vi "Find PS3 Controller.vi"(8 "error in (no error)":errorcluster) -> (0 "error out":errorcluster, 2 "Index_out":u64, 3 "Controller Reference Out":refnum<k1>)   [LabVIEW 2024]
doc: "This VI finds the first DualShock 3 controller identified by the operating system as a Joystick."
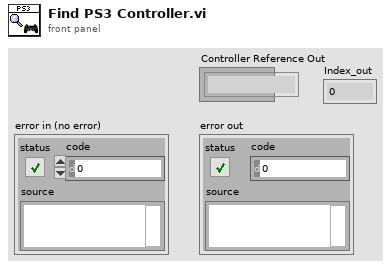
[diagram p1: front panel]
types:
  T1 = cluster{"axes total":u32, "buttons total":u32, "pov total":u32, "device name":string}[]
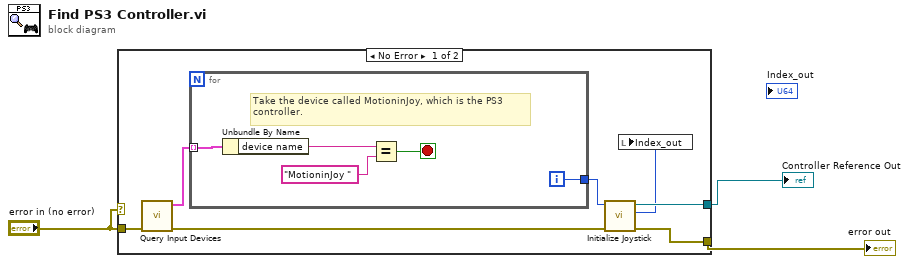
[diagram p0: block diagram]
diagram:
  n1 = case shown="No Error" "error in (no error)" {
    tunnel: "error in (no error)" -> [w10 w16]
    tunnel: [w7 _] -> w3
    tunnel: [w6 w16] -> w2
    frame No Error {
      n2 = call <vilib>:"Query Input Devices.vi"("error in (no error)"=w10) -> ("error out"=w5:errorcluster, "joystick info"=w8:T1)  [unwired: 9 out]
      n3 = for {
        tunnel: w8 -> [w15] mode=indexing
        tunnel: [w11] -> w9
        i -> [w11]
        stop <- w12 stop-if-true
        # "Take the device called MotioninJoy, which is the PS3 controller."
        n4 = Unbundle By Name(w15) -> ("device name"=w14:string)
        n5 = Equal?(x=w14, y="MotioninJoy ") -> (x = y?=w12:bool)
      }
      n6 = call <vilib>:"Initialize Joystick.vi"("error in (no error)"=w5, "device index"=w9) -> ("error out"=w6:errorcluster, "Index_out"=w4:u64, "device ID"=w7:refnum<k1>)  [unwired: 7 out]
      n7 = local write "Index_out"(w4) -> ()
    }
    frame Error {
    }
  }
  "Controller Reference Out" <- w3
  "error out" <- w2
